vi "Test Addressing Correct for Address 2.vi"(11 "Test Case In":refnum<class "MCP23017 Test.lvclass">) -> (0 "error out":errorcluster, 3 "Test Case Out":refnum<class "MCP23017 Test.lvclass">)   [LabVIEW 2020, in "MCP23017 Test.lvclass"]
uses:
  MCP23017 Test.lvclass
  C:/Program Files (x86)/National Instruments/LabVIEW 2020/vi.lib/Astemes/LUnit/Test Case.lvclass
  Mock I2C Bus/Mock I2C Bus.lvclass
  C:/Program Files (x86)/National Instruments/LabVIEW 2020/vi.lib/Astemes/LMock/Mock.lvclass
  C:/git/astemes-mocking-exercise/source/I2C Bus Interface/I2C Bus.lvclass
  <vilib>/Astemes/LMock/One Identical Inputs.vi
  <vilib>/Astemes/LMock/LMock Verifier.lvclass
  <vilib>/Astemes/LMock/LMock.lvlib
  C:/git/astemes-mocking-exercise/tests/Mock I2C Bus/Mock I2C Bus.lvclass
  source/MCP23017/MCP23017.lvclass
  <vilib>/Astemes/LMock/LMock One.lvlib
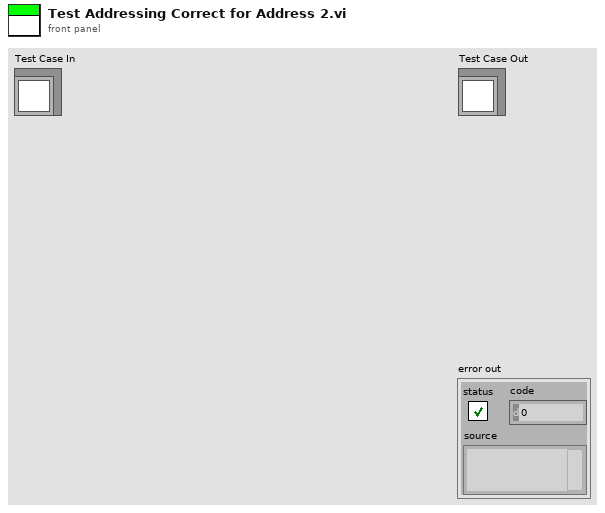
[diagram p1: front panel]
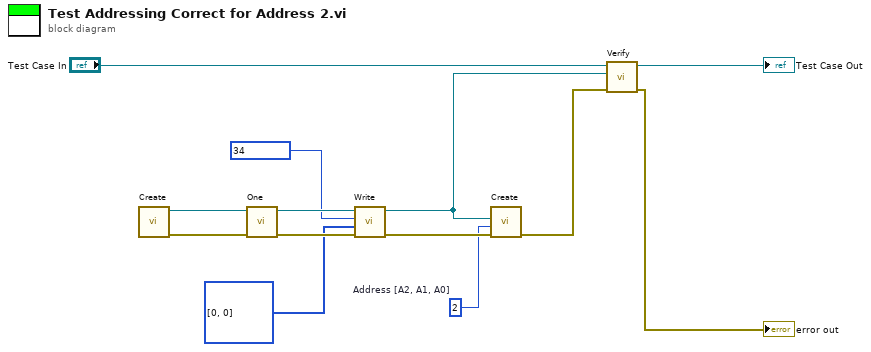
[diagram p0: block diagram]
diagram:
  w1 = u8 2  # Address [A2, A1, A0]
  n1 = call "Create.vi"() -> ("error out"=w10:errorcluster, "Mock Class Generator out"=w8:refnum<class "Mock I2C Bus.lvclass">)  [unwired: 10 in]
  n2 = call-poly <vilib>:"One.vi"("error in (no error)"=w10, "Mock in"=w8) -> ("error out"=w9:errorcluster, "Mock out"=w7:refnum<class "Mock I2C Bus.lvclass">)  [unwired: 8 in]
  n3 = call-dynamic "Write.vi"("error in (no error)"=w9, "Data"=u8[] [0, 0], "Address"=u8 34, "I2C Bus In"=w7) -> ("error out"=w4:errorcluster, "I2C Bus Out"=w2:refnum<class "Mock I2C Bus.lvclass">)  [unwired: 6 in]
  n4 = call "Create.vi"("error in (no error)"=w4, "Address [A2, A1, A0]"=w1, "I2C Bus"=w2) -> ("error out"=w3:errorcluster)  [unwired: 7 in, 1 out]
  n5 = call <vilib>:"Verify.vi"("error in (no error)"=w3, "Mock"=w2, "LUnit Test Case In"="Test Case In") -> ("error out"=→"error out":errorcluster, "LUnit Test Case Out"=→"Test Case Out":refnum<class "MCP23017 Test.lvclass">)  [unwired: 7 in]
